vi "RESTful Configure Service Attribute Settings.vi"(6 "Service Attribute Number (1..N)":i32, 8 "error in":errorcluster, 9 "RESTful service attribute":T1={"Name"="", "Service Attribute Type"=enum."Path", "Value"=""}, 10 "AMQP Ini In":string="#Service Attributes", 11 "Master Text In":string="#Service Attributes") -> (0 "error out":errorcluster, 2 "AMQP Ini Out":string="#Service Attributes", 3 "Master Text Out":string="#Service Attributes")   [LabVIEW 2020]
doc: "This VI configures the routing templates section of the webservices INI file."
uses:
  <vilib>/AppBuilder/AB_Classes/RESTful/AB_RESTful_ServiceAttribute.ctl
  <vilib>/AppBuilder/AB_Classes/RESTful/AB_RESTful_ServiceAttributeType.ctl
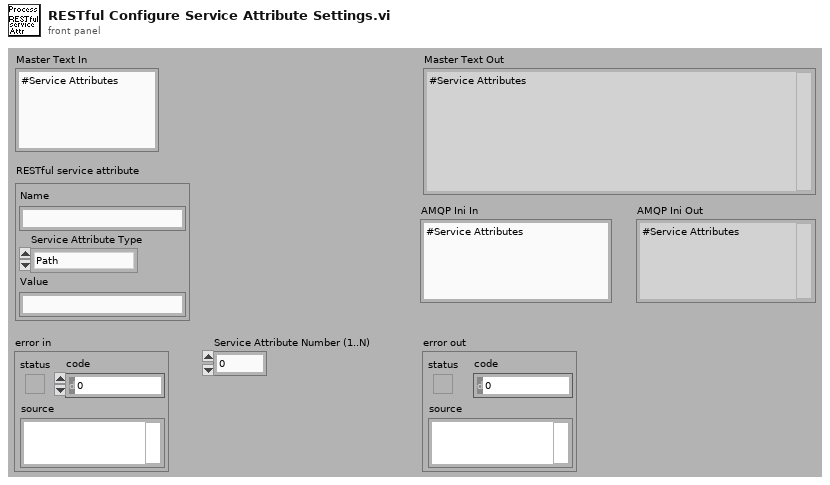
[diagram p1: front panel]
types:
  T1 = typedef "AB_RESTful_ServiceAttribute.ctl" = cluster{"Name":string, "Service Attribute Type":T2, "Value":string}
  T2 = typedef "AB_RESTful_ServiceAttributeType.ctl" = enum32{"String", "Path"}
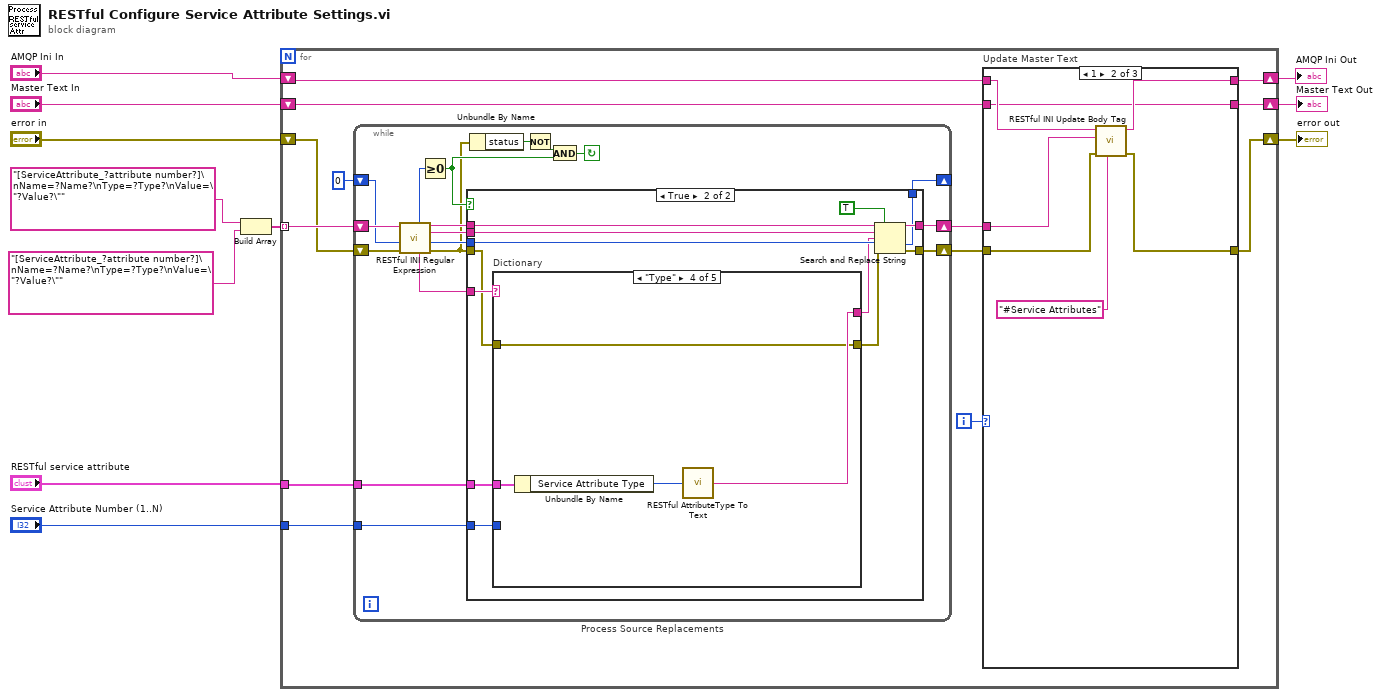
[diagram p0: block diagram]
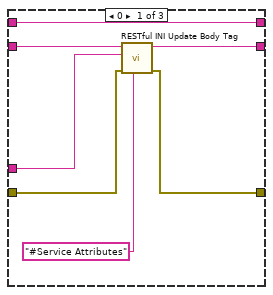
[diagram p2: hidden frame]
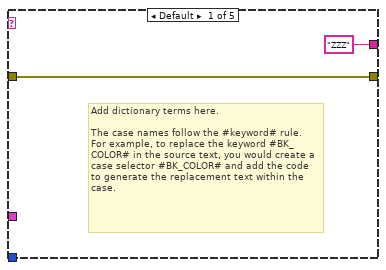
[diagram p5: hidden frame]
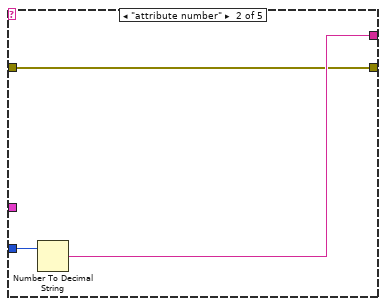
[diagram p6: hidden frame]
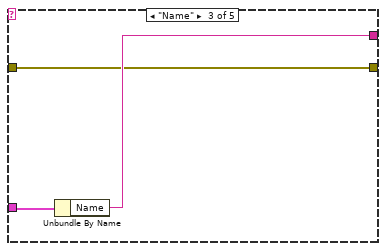
[diagram p7: hidden frame]
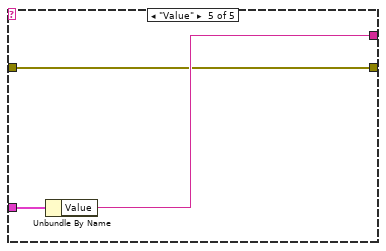
[diagram p8: hidden frame]
diagram:
  n1 = Build Array("[ServiceAttribute_?attribute number?]\nName=?Name?\nType=?Type?\nValue=\"?Value?\"", "[ServiceAttribute_?attribute number?]\nName=?Name?\nType=?Type?\nValue=\"?Value?\"") -> (w3:string[])
  n2 = for {
    tunnel: w3 -> [w24] mode=indexing
    shift-right: [w21] -> w10
    shift-left: "Master Text In" -> [w22]
    shift-right: [w18] -> w9
    shift-left: "error in" -> [w20]
    tunnel: "RESTful service attribute" -> [w15]
    tunnel: "Service Attribute Number (1..N)" -> [w14]
    shift-right: [w12] -> w4
    shift-left: "AMQP Ini In" -> [w13]
    i -> [w23]
    n3 = while "Process Source Replacements" {
      shift-right: [w54] -> w17
      shift-left: w24 -> [w59]
      shift-right: [w52] -> w19
      shift-left: w20 -> [w53]
      shift-right: [w51] -> _
      shift-left: 0 ("offset past replacement") -> [w50]
      tunnel: w15 -> [w43]
      tunnel: w14 -> [w42]
      stop <- w46 continue-if-true
      n4 = call <vilib>:"RESTful INI Regular Expression.vi"("error in"=w53, "offset (0)"=w50, "input string"=w59) -> ("error out"=w47:errorcluster, "Offset of match"=w56:i32, "whole match"=w55:string, "dup input string"=w57:string, "keyword"=w48:string, "offset past match"=w58:i32)  [unwired: 3 out]
      n5 = Greater Or Equal To 0?(x=w58) -> (x >= 0?=w49:bool)
      n6 = case shown="True" w49 {
        tunnel: w57 -> [w62 w75]
        tunnel: w56 -> [w60 w74]
        tunnel: w55 -> [_ w73]
        tunnel: [w62 w72] -> w54
        tunnel: [w61 w71] -> w52
        tunnel: w47 -> [w61 w68]
        tunnel: [w60 w70] -> w51
        tunnel: w48 -> [_ w69]
        tunnel: w43 -> [_ w66]
        tunnel: w42 -> [_ w65]
        frame False {
        }
        frame True {
          n7 = case "Dictionary" shown="\"Type\"" w69 {
            tunnel: w68 -> [w77 w78 w81 w84 w88]
            tunnel: [w77 w78 w81 w84 w88] -> w67
            tunnel: w66 -> [_ _ w83 w87 w90]
            tunnel: w65 -> [_ w80 _ _ _]
            tunnel: ["ZZZ" w79 w82 w85 w89] -> w64
            frame Default {
              # "Add dictionary terms here.\n\nThe case names follow the #keyword# rule.  For example, to replace the keyword #BK_COLOR# in the source text, you would create a case selector #BK_COLOR# and add the code to generate the replacement text within the case."
            }
            frame "attribute number" {
              n8 = Number To Decimal String(number=w80) -> (decimal integer string=w79:string)  [unwired: 1 out]
            }
            frame "Name" {
              n9 = Unbundle By Name(w83) -> ("Name"=w82:string)
            }
            frame "Type" {
              n10 = Unbundle By Name(w87) -> ("Service Attribute Type"=w86:T2)
              n11 = call <vilib>:"RESTful AttributeType To Text.vi"("Service Attribute Type"=w86) -> ("Boolean Text"=w85:string)
            }
            frame "Value" {
              n12 = Unbundle By Name(w90) -> ("Value"=w89:string)
            }
          }
          n13 = Search and Replace String(replace all?=TRUE ("replace all? (F)"), input string=w75, search string=w73, replace string=w64, offset=w74, error in=w67) -> (result string=w72:string, offset past replacement=w70:i32, error out=w71:errorcluster)  [unwired: 3 out]
        }
      }
      n14 = Unbundle By Name(w47) -> ("status"=w45:bool)
      n15 = Not(x=w45) -> (.not. x?=w44:bool)
      n16 = And(x=w44, y=w49) -> (x .and. y?=w46:bool)
    }
    n17 = case "Update Master Text" shown="1" w23 {
      tunnel: w22 -> [w31 w32 w41]
      tunnel: [w30 w32 w41] -> w21
      tunnel: w19 -> [w28 w37 w40]
      tunnel: [w27 w36 w40] -> w18
      tunnel: w17 -> [w29 w38 _]
      tunnel: w13 -> [w25 w34 w39]
      tunnel: [w25 w33 w39] -> w12
      frame 0 {
        n18 = call <vilib>:"RESTful INI Update Body Tag.vi"("Tag"="#Service Attributes", "error in (no error)"=w28, "Replacement String"=w29, "Input String"=w31) -> ("error out"=w27:errorcluster, "result string"=w30:string)  [unwired: 6 out]
      }
      frame 1 {
        n19 = call <vilib>:"RESTful INI Update Body Tag.vi"("Tag"="#Service Attributes", "error in (no error)"=w37, "Replacement String"=w38, "Input String"=w34) -> ("error out"=w36:errorcluster, "result string"=w33:string)  [unwired: 6 out]
      }
      frame Default {
      }
    }
  }
  "error out" <- w9
  "Master Text Out" <- w10
  "AMQP Ini Out" <- w4
